vi "Utility - Detect Modules.vi"(8 "error in (no error)":errorcluster caption="错误输入（无错误）", 11 "Controller IP":string="localhost" caption="控制器IP") -> (0 "error out":errorcluster caption="错误输出", 3 "cRIO 9074":string[](array[string]) caption="模块列表")   [LabVIEW 2015]
uses:
  <resource>/objmgr/cRIO.rc
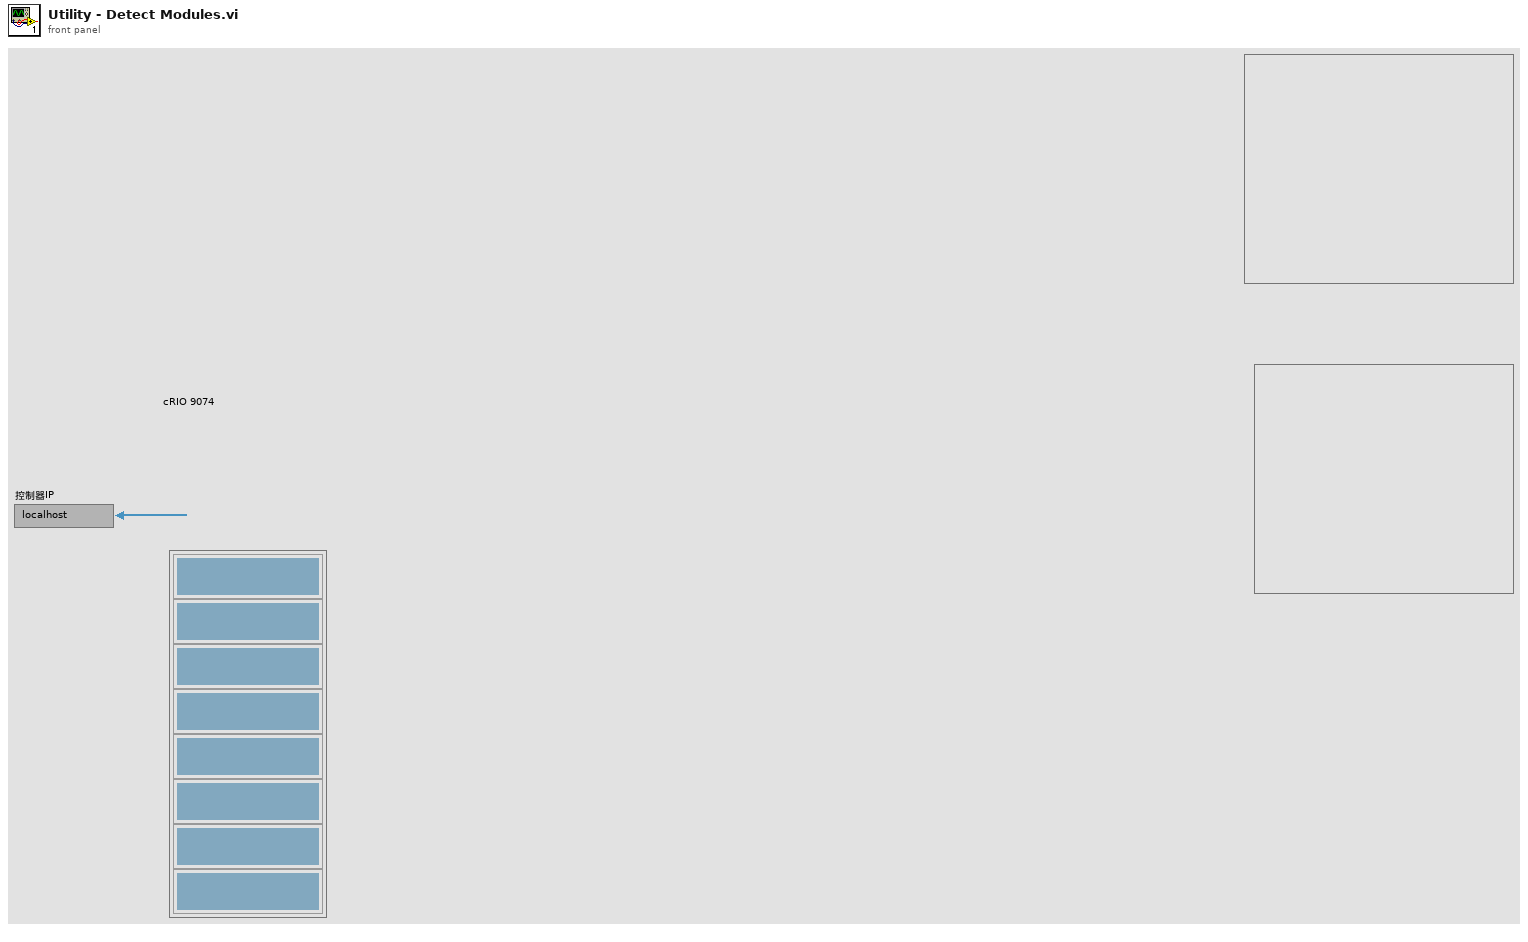
[diagram p1: front panel]
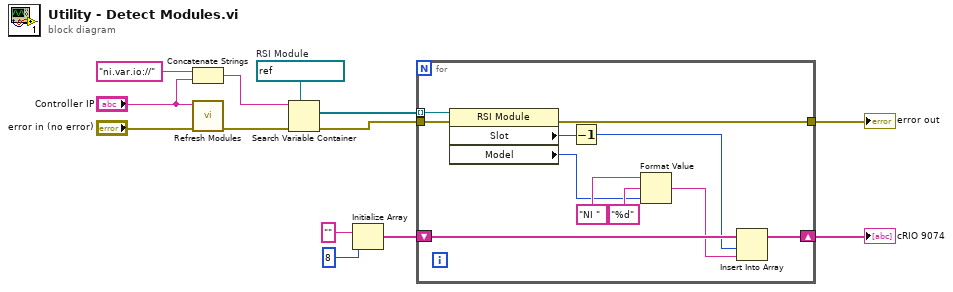
[diagram p0: block diagram]
diagram:
  w13 = refnum<k21> refnum  # RSI Module
  n1 = Concatenate Strings("ni.var.io://", "Controller IP") -> (w9:string)
  n2 = call <vilib>:"Refresh Modules.vi"("error in (no error)"="error in (no error)", "target address (localhost)"="Controller IP") -> ("error out"=w12:errorcluster)  [unwired: 9 in]
  n3 = Search Variable Container(7:w13, 8:w12, 11:w9) -> (0:w3:errorcluster, 2:w10:refnum<k21>[])  [unwired: 3 in, 1 out]
  n4 = Initialize Array("", 8 ("维数大小")) -> (w4:string[])
  n5 = for {
    tunnel: w10 -> [w24] mode=indexing
    shift-right: [w22] -> w7
    shift-left: w4 -> [w23]
    tunnel: w3 -> [w17]
    tunnel: [w15] -> w1
    n6 = property class="RSI Module"(reference=w24, error in=w17) -> (error out=w15:errorcluster, "Slot"=w16:u32, "Model"=w14:u32)  [unwired: 1 out]
    n7 = Decrement(x=w16) -> (x-1=w20:u32)
    n8 = Format Value(string ("")="NI ", format string="%d" ("格式字符串"), value (0)=w14) -> (output string=w21:string)
    n9 = Insert Into Array(array=w23, index=w20, new element=w21) -> (w22:string[])
  }
  "cRIO 9074" <- w7
  "error out" <- w1
